vi "Instr Initialize.vi"(8 "error in":errorcluster, 10 "Device \n(Case Sensitive)":string="Report", 11 "Application Directory":path) -> (0 "error out":errorcluster, 3 "Report out":refnum<class "Report.lvclass">)   [LabVIEW 2019, in "Report.lvlib" / "Report.lvclass"]
uses:
  Report.lvclass
  C:/Users/rdexter/Documents/Development/Drivers/PPL/Instruments.lvlibp/Instruments.lvclass
  PPL/Instruments.lvlibp/Instruments.lvclass
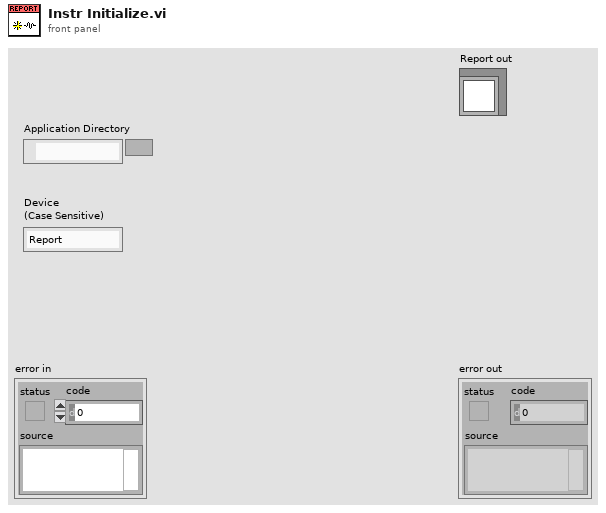
[diagram p1: front panel]
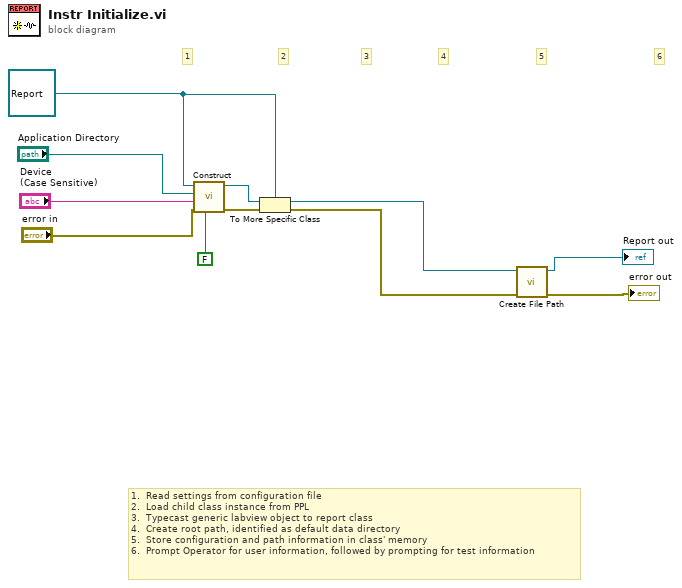
[diagram p0: block diagram]
diagram:
  w10 = refnum<class "Report.lvclass"> refnum ("Report in")
  # "6"
  # "5"
  # "4"
  # "1.  Read settings from configuration file\n2.  Load child class instance from PPL\n3.  Typecast generic labview object to report class\n4.  Create root path, identified as default data directory\n5.  Store configuration and path information in class' memory\n6.  Prompt Operator for user information, followed by prompting for test information"
  # "3"
  # "2"
  # "1"
  n1 = call "Construct.vi"("Scripting"=FALSE, "error in (no error)"="error in", "Handle"="Device \n(Case Sensitive)", "Application Directory"="Application Directory", "Instruments in"=w10) -> ("error out"=w9:errorcluster, "Instruments out"=w11:refnum<class "Instruments.lvclass">)  [unwired: 5 in]
  n2 = To More Specific Class(target class=w10, reference=w11, error in=w9) -> (specific class reference=w1:refnum<class "Report.lvclass">, error out=w4:errorcluster)
  n3 = call "Create File Path.vi"("error in"=w4, "Report in"=w1) -> ("error out"=→"error out":errorcluster, "Report out"=→"Report out":refnum<class "Report.lvclass">)  [unwired: 8 in]
